vi "Interact.vi"(0 "subprocess in":refnum<class "Subprocess.lvclass">, 1 "stdin buffer":u8[](array[numeric]) format="%02x", 2 "read size":i32, 5 "error in":errorcluster, 6 "select stdin":bool=TRUE, 7 "deadline":T1={"mode"=enum."Relative", "deadline (ms)"=30000}, 8 "select stdout":bool=TRUE, 10 "select stderr":bool=TRUE) -> (11 "stdout eof?":bool, 13 "stderr eof?":bool, 14 "subprocess out":refnum<class "Subprocess.lvclass">, 15 "stdin written":i32, 16 "stdout buffer out":u8[](array[numeric]) format="%02x", 17 "stderr buffer out":u8[](array[numeric]) format="%02x", 19 "error out":errorcluster)   [LabVIEW 2020, in "NI_Subprocess.lvlib" / "Subprocess.lvclass"]
uses:
  <vilib>/Subprocess/Subprocess/Subprocess.lvclass
  <vilib>/Utility/Deadline/Deadline.ctl
  <vilib>/Utility/Deadline/Mode.ctl
  <vilib>/Subprocess/Subprocess/Subprocess.lvclass/Subprocess.ctl
  <vilib>/Utility/Deadline/NI_Deadline.lvlib
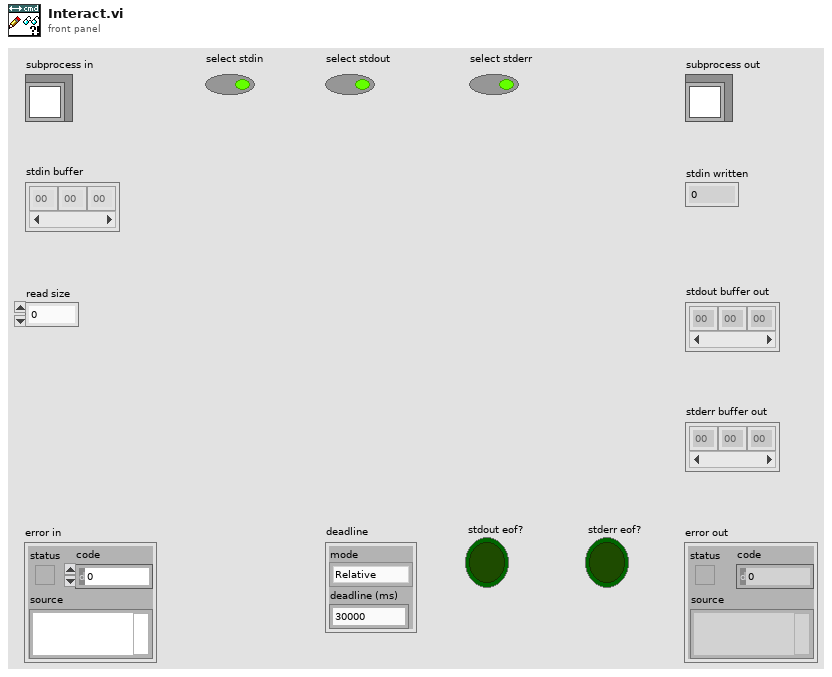
[diagram p1: front panel]
types:
  T1 = typedef "NI_Deadline.lvlib/Deadline.ctl" = cluster{"mode":T2, "deadline (ms)":u32}
  T2 = typedef "NI_Deadline.lvlib/Mode.ctl" = enum16{"Relative", "Use deadline", "Wait forever", "Nonblocking", "N/A"}
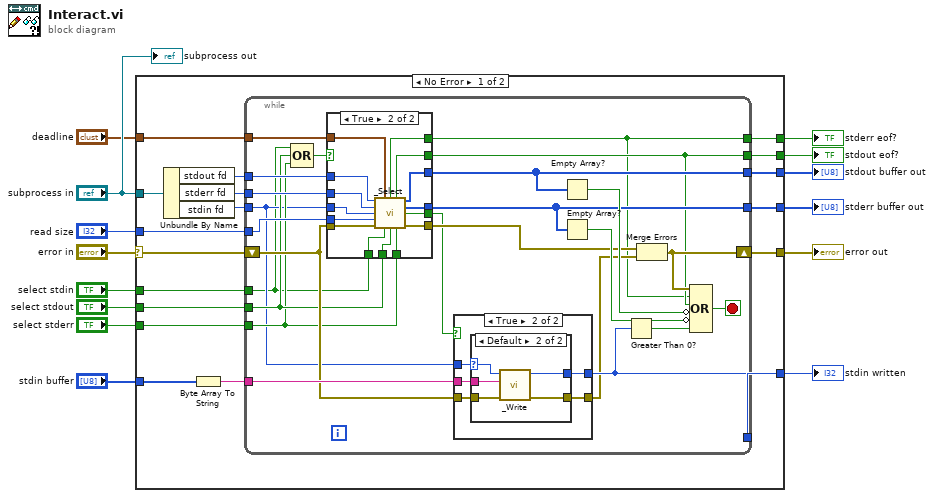
[diagram p0: block diagram]
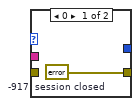
[diagram p3: hidden frame]
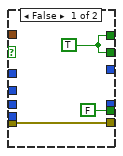
[diagram p4: hidden frame]
diagram:
  n1 = case shown="No Error" "error in" {
    selector: "error in" -> [w32 w87]
    tunnel: [w17 w87] -> w13
    tunnel: "subprocess in" -> [w18 _]
    tunnel: "select stdin" -> [w31 _]
    tunnel: "select stdout" -> [w30 _]
    tunnel: "select stderr" -> [w29 _]
    tunnel: "stdin buffer" -> [w28 _]
    tunnel: [w27 _] -> w9
    tunnel: "read size" -> [w26 _]
    tunnel: [w25 _] -> w8
    tunnel: [w22 _] -> w6
    tunnel: [w24 _] -> w5
    tunnel: [w23 _] -> w4
    tunnel: "deadline" -> [w16 _]
    frame No Error {
      n2 = Unbundle By Name(w18) -> ("stdout fd"=w19:u64, "stderr fd"=w21:u64, "stdin fd"=w15:u64)
      n3 = Byte Array To String(unsigned byte array=w28) -> (string=w20:string)
      n4 = while {
        shift-right: [w41] -> w17
        shift-left: w32 -> [w44]
        tunnel: w31 -> [w33]
        tunnel: w30 -> [w37]
        tunnel: w29 -> [w36]
        tunnel: w20 -> [w56]
        tunnel: [w55] -> w27
        tunnel: w26 -> [w53]
        tunnel: [w50] -> w25
        tunnel: [w39] -> w24
        tunnel: [w38] -> w23
        tunnel: [w43] -> w22
        tunnel: w21 -> [w54]
        tunnel: w19 -> [w52]
        tunnel: w16 -> [w42]
        tunnel: w15 -> [w35]
        stop <- w40 stop-if-true
        n5 = Compound Arithmetic op=OR(w33, w37, w36) -> (w51:bool)
        n6 = case shown="True" w51 {
          tunnel: w52 -> [_ w86]
          tunnel: w44 -> [w71 w85]
          tunnel: [w71 w80] -> w45
          tunnel: w53 -> [_ w76]
          tunnel: [_ w81] -> w50
          tunnel: [w70 w82] -> w39
          tunnel: w54 -> [_ w84]
          tunnel: [_ w83] -> w43
          tunnel: [w70 w79] -> w38
          tunnel: w42 -> [_ w75]
          tunnel: w37 -> [_ w78]
          tunnel: w36 -> [_ w77]
          tunnel: w35 -> [_ w74]
          tunnel: w33 -> [_ w73]
          tunnel: [FALSE ("stdin ready?") w72] -> w34
          frame False {
            w70 = TRUE ("eof?")
          }
          frame True {
            n7 = call <vilib>:"_Select.vi"("stdout fd"=w86, "deadline"=w75, "stderr fd"=w84, "stdin fd"=w74, "read size"=w76, "error in (no error)"=w85, "select stdin"=w73, "select stdout"=w78, "select stderr"=w77) -> ("stderr eof?"=w79:bool, "stdout eof?"=w82:bool, "stdout data"=w81:u8[], "stderr data"=w83:u8[], "stdin ready?"=w72:bool, "error out"=w80:errorcluster)  [unwired: 1 in]
          }
        }
        n8 = case shown="True" w34 {
          tunnel: w44 -> [w57 w62]
          tunnel: w56 -> [_ w60]
          tunnel: w35 -> [_ w59]
          tunnel: [w57 w61] -> w46
          tunnel: [_ w58] -> w55
          frame False {
          }
          frame True {
            n9 = case shown="Default" w59 {
              selector: w59 -> [_ w66]
              tunnel: w62 -> [_ w67]
              tunnel: [w63 w68] -> w61
              tunnel: w60 -> [_ w65]
              tunnel: [_ w64] -> w58
              frame 0 {
                w63 = errorcluster {"status"=TRUE, "code"=-917, "source"=""}  # -917: session closed
              }
              frame Default {
                n10 = call <vilib>:"_Write.vi"("error in (no error)"=w67, "data"=w65, "file descriptor"=w66) -> ("error out"=w68:errorcluster, "written"=w64:i32)  [unwired: 7 in]
              }
            }
          }
        }
        n11 = Empty Array?(array=w50) -> (empty?=w49:bool)
        n12 = Empty Array?(array=w43) -> (empty?=w48:bool)
        n13 = Greater Than 0?(x=w55) -> (x > 0?=w47:bool)
        n14 = Merge Errors(w45, w46) -> (w41:errorcluster)
        n15 = Compound Arithmetic op=OR(w41, w38, w39, invert w49, invert w48, w47) -> (w40:bool)
      }
    }
    frame Error {
    }
  }
  "error out" <- w13
  "stdout buffer out" <- w8
  "stdout eof?" <- w5
  "stderr eof?" <- w4
  "stderr buffer out" <- w6
  "stdin written" <- w9
  "subprocess out" <- "subprocess in"
